vi "globalreport.vi"() -> ()   [LabVIEW 2012]
panel:
  in  "test report":T1(array[cluster])
  in  "report":T2(array[cluster])
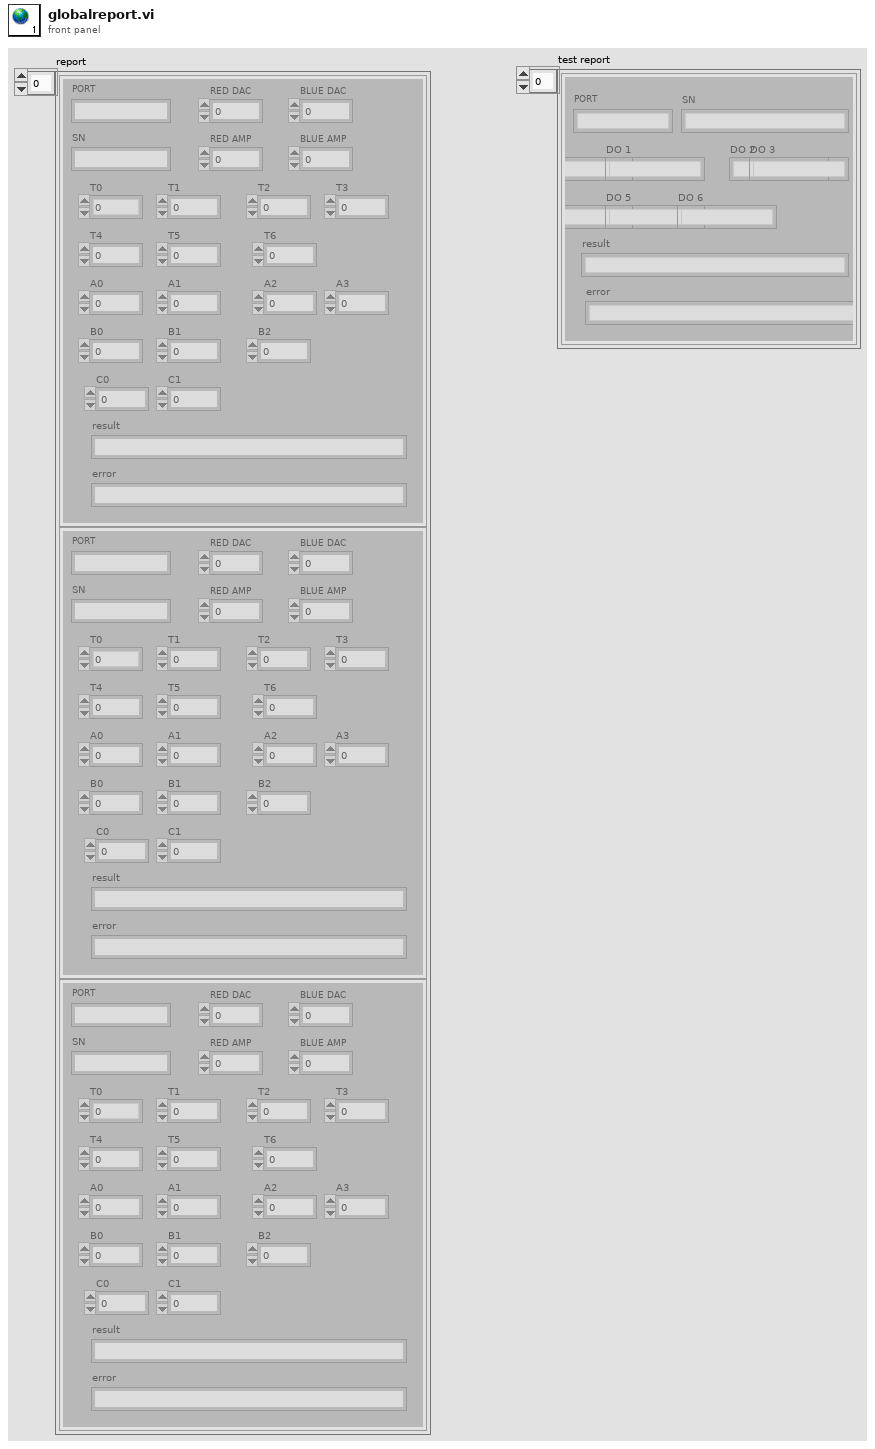
[diagram p1: front panel]
types:
  T1 = cluster{"PORT":string, "SN":string, "DO 0":string, "DO 1":string, "DO 2":string, "DO 3":string, "DO 4":string, "DO 5":string, "DO 6":string, "result":string, "error":string}[]
  T2 = cluster{"PORT":string, "SN":string, "RED DAC":dbl, "BLUE DAC":dbl, "RED AMP":dbl, "BLUE AMP":dbl, "T0":dbl, "T1":dbl, "T2":dbl, "T3":dbl, "T4":dbl, "T5":dbl, "T6":dbl, "A0":dbl, "A1":dbl, "A2":dbl, "A3":dbl, "B0":dbl, "B1":dbl, "B2":dbl, "C1":dbl, "C0":dbl, "result":string, "error":string}[]
diagram:
